vi "ir_laser_test.vi"() -> ()   [LabVIEW 2009]
uses:
  <vilib>/Utility/error.llb/DialogType.ctl
  <vilib>/DAQmx/read.llb/DAQmx Read (Analog 2D DBL NChan NSamp).vi
  <vilib>/DAQmx/write.llb/DAQmx Write (Analog 1D DBL 1Chan NSamp).vi
  <vilib>/DAQmx/configure/timing.llb/DAQmx Timing (Sample Clock).vi
  <vilib>/DAQmx/create/channels.llb/DAQmx Create Channel (AO-Voltage-Basic).vi
  <vilib>/DAQmx/create/channels.llb/DAQmx Create Channel (AI-Voltage-Basic).vi
  <vilib>/Utility/file.llb/Write To Spreadsheet File (DBL).vi
  <vilib>/Analysis/NI_AALBase.lvlib
panel:
  out "Current laser power [W]":dbl
  in  "Amplitudes [W]":dbl[](array[numeric])
  in  "repetitions":i32=3
  in  "Save file":bool
  in  "filename":path
  out "Laser [W]":dbl[](graph) caption="Laser control"
  out "Temperature":dbl[](graph)
  out "Current [pA]":dbl[](graph) caption="Current"
  in  "Recording  duration":dbl=10.0 caption="Duration [s]" format="%0.2p"
  in  "Pulse duration":dbl=1.0 caption="Pulse duration [s]" format="%0.2p"
  in  "Amplitude":dbl=1.0 caption="Amplitude [W]" format="%0.2p"
  out "Measurement":dbl[][](graph)
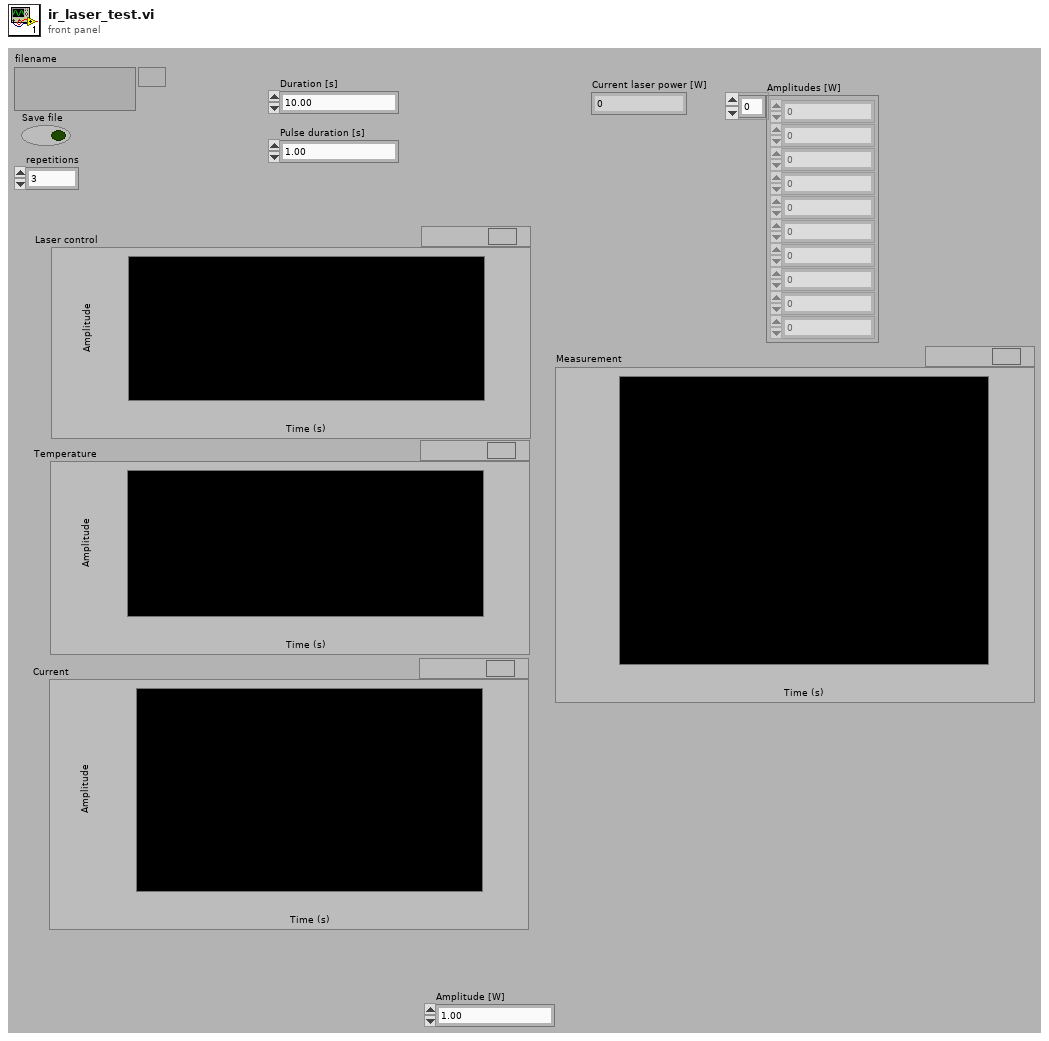
[diagram p1: front panel]
types:
  T1 = typedef "DialogType.ctl" = u16
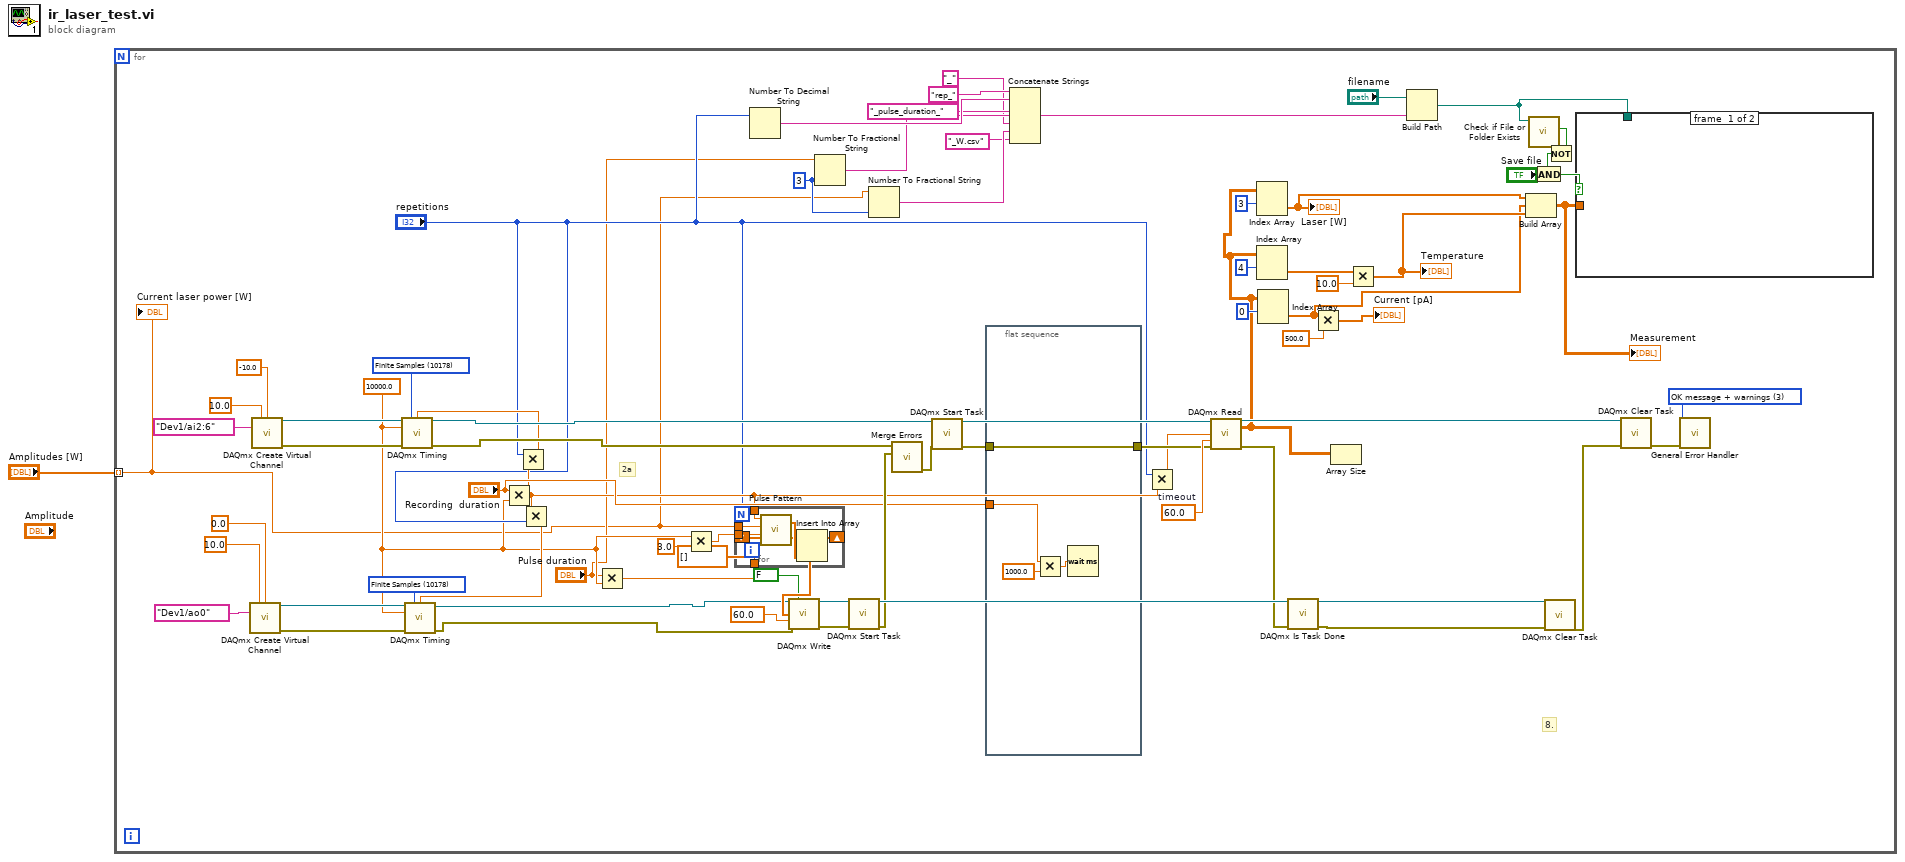
[diagram p0: block diagram]
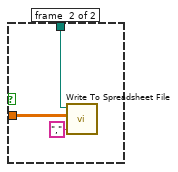
[diagram p2: hidden frame]
diagram:
  n1 = for {
    tunnel: "Amplitudes [W]" -> [w2] mode=indexing
    w12 = i16 3 ("precision (6)")
    w49 = 60.0  # timeout
    w13 = 10000.0 ("Rate")
    w60 = T1 3 items=["no dialog", "OK message", "continue or stop message", "OK message + warnings", "continue/stop + warnings"] ("type of dialog (OK msg:1)")
    w67 = 10178 items=["Finite Samples"=10178, "Continuous Samples"=10123] ("sample mode")
    w73 = 10178 items=["Finite Samples"=10178, "Continuous Samples"=10123] ("sample mode")
    # "2a"
    # "8."
    n2 = call-poly <vilib>:"DAQmx Create Virtual Channel.vi"("maximum value"=10.0, "minimum value"=0.0, "physical channels"=tag "Dev1/ao0") -> ("task out"=w66:refnum<k21>, "error out"=w65:errorcluster)  [unwired: 11 in]
    n3 = call-poly <vilib>:"DAQmx Create Virtual Channel.vi"("maximum value"=10.0 ("Maximum Value"), "minimum value"=-10.0 ("Minimum Value"), "physical channels"=tag "Dev1/ai2:6" ("Physical Channel")) -> ("task out"=w71:refnum<k21>, "error out"=w72:errorcluster)  [unwired: 11 in]
    n4 = Multiply(x="Recording  duration", y=w13) -> (x*y=w26:dbl)
    n5 = Multiply(x="repetitions", y=w26) -> (x*y=w18:dbl)
    n6 = call-poly <vilib>:"DAQmx Timing.vi"("task/channels in"=w71, "sample mode"=w73, "samples per channel"=w18, "rate"=w13, "error in"=w72) -> ("task out"=w30:refnum<k21>, "error out"=w31:errorcluster)  [unwired: 9 in]
    n7 = Multiply(x=w26, y="repetitions") -> (x*y=w19:dbl)
    n8 = call-poly <vilib>:"DAQmx Timing.vi"("task/channels in"=w66, "sample mode"=w67, "samples per channel"=w19, "rate"=w13, "error in"=w65) -> ("task out"=w28:refnum<k21>, "error out"=w29:errorcluster)  [unwired: 9 in]
    n9 = Multiply(x="Pulse duration", y=w13) -> (x*y=w52:dbl)
    n10 = Multiply(x=w13, y=3.0) -> (x*y=w50:dbl)
    n11 = for {
      N: "repetitions" -> [_]
      tunnel: w2 -> [w83]
      tunnel: w52 -> [w82]
      tunnel: w50 -> [w81]
      tunnel: w26 -> [w80]
      shift-right: [w79] -> w37
      shift-left: dbl[] [] -> [w77]
      n12 = call <vilib>:"Pulse Pattern.vi"("width"=w82, "delay"=w81, "amplitude"=w83, "samples"=w80) -> ("Pulse Pattern"=w78:dbl[])  [unwired: 1 out]
      n13 = Insert Into Array(array=w77, new element=w78) -> (w79:dbl[])  [unwired: 1 in]
    }
    n14 = Number To Decimal String(number="repetitions") -> (decimal integer string=w10:string)  [unwired: 1 in]
    n15 = call-poly <vilib>:"DAQmx Write.vi"("task/channels in"=w28, "auto start"=FALSE, "data"=w37, "timeout"=60.0 ("Wirite Timeout"), "error in"=w29) -> ("task out"=w62:refnum<k21>, "error out"=w61:errorcluster)  [unwired: 8 in, 1 out]
    n16 = Number To Fractional String(number="Pulse duration", precision (6)=w12) -> (F-format string=w8:string)  [unwired: 2 in]
    n17 = call <vilib>:"DAQmx Start Task.vi"("task/channels in"=w62, "error in"=w61) -> ("task out"=w64:refnum<k21>, "error out"=w57:errorcluster)  [unwired: 12 in]
    n18 = Number To Fractional String(number=w2, precision (6)=w12) -> (F-format string=w6:string)  [unwired: 2 in]
    n19 = call <vilib>:"Merge Errors.vi"("error in 2 (no error)"=w57, "error in 1 (no error)"=w31) -> ("error out"=w56:errorcluster)  [unwired: 5 in]
    n20 = call <vilib>:"DAQmx Start Task.vi"("task/channels in"=w30, "error in"=w56) -> ("task out"=w58:refnum<k21>, "error out"=w39:errorcluster)  [unwired: 12 in]
    n21 = flat-sequence {
      tunnel: w39 -> [w90]
      tunnel: [w90] -> w38
      tunnel: "Recording  duration" -> [w89]
      frame #0 {
        n22 = Multiply(x=w89, y=1000.0) -> (x*y=w88:dbl)
        n23 = Wait (ms)(milliseconds to wait=w88) -> ()  [unwired: 1 out]
      }
    }
    n24 = Concatenate Strings("rep_" ("string"), w10, "_pulse_duration_" ("string"), w8, "_" ("string"), w6, "_W.csv" ("format string")) -> (w4:string)
    n25 = Multiply(x="repetitions", y=w26) -> (x*y=w17:dbl)
    n26 = call-poly <vilib>:"DAQmx Read.vi"("task/channels in"=w58, "number of samples per channel"=w17, "timeout"=w49, "error in"=w38) -> ("task out"=w74:refnum<k21>, "data"=w42:dbl[][], "error out"=w48:errorcluster)  [unwired: 9 in]
    n27 = Index Array(array=w42, index (row)=3) -> (element=w35:dbl[])  [unwired: 1 in]
    "Laser [W]" <- w35
    n28 = Index Array(array=w42, index (row)=4) -> (element=w46:dbl[])  [unwired: 1 in]
    n29 = Index Array(array=w42, index (row)=0) -> (element=w21:dbl[])  [unwired: 1 in]
    n30 = call <vilib>:"DAQmx Is Task Done.vi"("task/channels in"=w64, "error in"=w48) -> ("task out"=w63:refnum<k21>, "error out"=w55:errorcluster)  [unwired: 11 in, 1 out]
    n31 = Multiply(x=w21, y=500.0 ("Minimum Value")) -> (x*y=→"Current [pA]":dbl[])
    n32 = Array Size(array=w42) -> ()  [unwired: 1 out]
    n33 = Multiply(x=w46, y=10.0 ("Minimum Value")) -> (x*y=w33:dbl[])
    "Temperature" <- w33
    n34 = Build Path(base path="filename", name or relative path=w4) -> (appended path=w15:path)
    n35 = Build Array(w35, w21, w33) -> (w25:dbl[][])
    "Measurement" <- w25
    n36 = call <vilib>:"Check if File or Folder Exists.vi"("path"=w15) -> ("file or folder exists?"=w23:bool)  [unwired: 8 in, 2 out]
    n37 = call <vilib>:"DAQmx Clear Task.vi"("task in"=w63, "error in"=w55) -> ("error out"=w54:errorcluster)  [unwired: 13 in]
    n38 = Not(x=w23) -> (.not. x?=w22:bool)
    n39 = And(x=w22, y="Save file") -> (x .and. y?=w24:bool)
    n40 = case shown="True" w24 {
      tunnel: w25 -> [_ w86]
      tunnel: w15 -> [_ w84]
      frame #0 {
      }
      frame #1 {
        n41 = call-poly <vilib>:"Write To Spreadsheet File.vi"("delimiter (\\t)"="," ("delimiter (\\t)"), "2D data"=w86, "file path (dialog if empty)"=w84) -> ()  [unwired: 5 in, 1 out]
      }
    }
    n42 = call <vilib>:"DAQmx Clear Task.vi"("task in"=w74, "error in"=w54) -> ("error out"=w53:errorcluster)  [unwired: 13 in]
    n43 = call <vilib>:"General Error Handler.vi"("type of dialog (OK msg:1)"=w60, "error in (no error)"=w53) -> ()  [unwired: 9 in, 5 out]
    "Current laser power [W]" <- w2
  }
